vi "Periodic Tasks.vi"(8 "error in":errorcluster) -> ()   [LabVIEW 2017]
doc: "This VI runs in parallel to other tasks. It can contain as many user-defined periodic loops as you need. These can carry out PID or other sorts of timed response."
uses:
  <vilib>/Rock Robotics/WPI/Utilities/WPI_GetSetVariantRefNum.vi
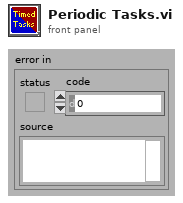
[diagram p1: front panel]
types:
  T1 = typedef "WPI_JoystickDevRef.ctl" = cluster{"Device":T2}
  T2 = typedef "WPI_JoystickDeviceEnum.ctl" = enum16{"USB 0", "USB 1", "USB 2", "USB 3", "USB 4", "USB 5"}
  T3 = typedef "WPI_MotorControlDeviceRef.ctl" = cluster{"DeviceStatus":errorcluster, "Type":T4, "PWM":cluster{"PWM Channel":T5, "DeadBand":T6}, "CAN":cluster{"Device Number":u8, "SetOutput VI Ref":variant, "GetOutput VI Ref":variant, "Enable VI Ref":variant, "Disable VI Ref":variant, "Data":variant}, "Invert":bool, "DIO PWM":cluster{"PWM \"Enable\" Channel":T5, "DIOChannel":T7, "PWM Rate":dbl}}
  T4 = typedef "WPI_MotorControlType.ctl" = enum16{"PWM", "CAN", "DIO PWM"}
  T5 = typedef "FPGA_DIOPWMChannel.ctl" = enum8{"PWM 0", "PWM 1", "PWM 2", "PWM 3", "PWM 4", "PWM 5", "PWM 6", "PWM 7", "PWM 8", "PWM 9", "PWM MXP 0", "PWM MXP 1", "PWM MXP 2", "PWM MXP 3", "PWM MXP 4", "PWM MXP 5", "PWM MXP 6", "PWM MXP 7", "PWM MXP 8", "PWM MXP 9", "Invalid"}
  T6 = typedef "WPI_PWMDeadband.ctl" = cluster{"Name":string, "maxPositivePwm":i32, "minPositivePwm":i32, "centerPwm":i32, "maxNegativePwm":i32, "minNegativePwm":i32, "angularRange":u16}
  T7 = typedef "FPGA_DIOChannel.ctl" = enum8{"DIO 0", "DIO 1", "DIO 2", "DIO 3", "DIO 4", "DIO 5", "DIO 6", "DIO 7", "DIO 8", "DIO 9", "DIO MXP 0", "DIO MXP 1", "DIO MXP 2", "DIO MXP 3", "DIO MXP 4", "DIO MXP 5", "DIO MXP 6", "DIO MXP 7", "DIO MXP 8", "DIO MXP 9", "DIO MXP 10", "DIO MXP 11", "DIO MXP 12", "DIO MXP 13", "DIO MXP 14", "DIO MXP 15", "SPI Port CS1", "SPI Port CS2", "SPI Port CS3", "SPI Port MISO", "SPI Port MOSI", "Invalid"}
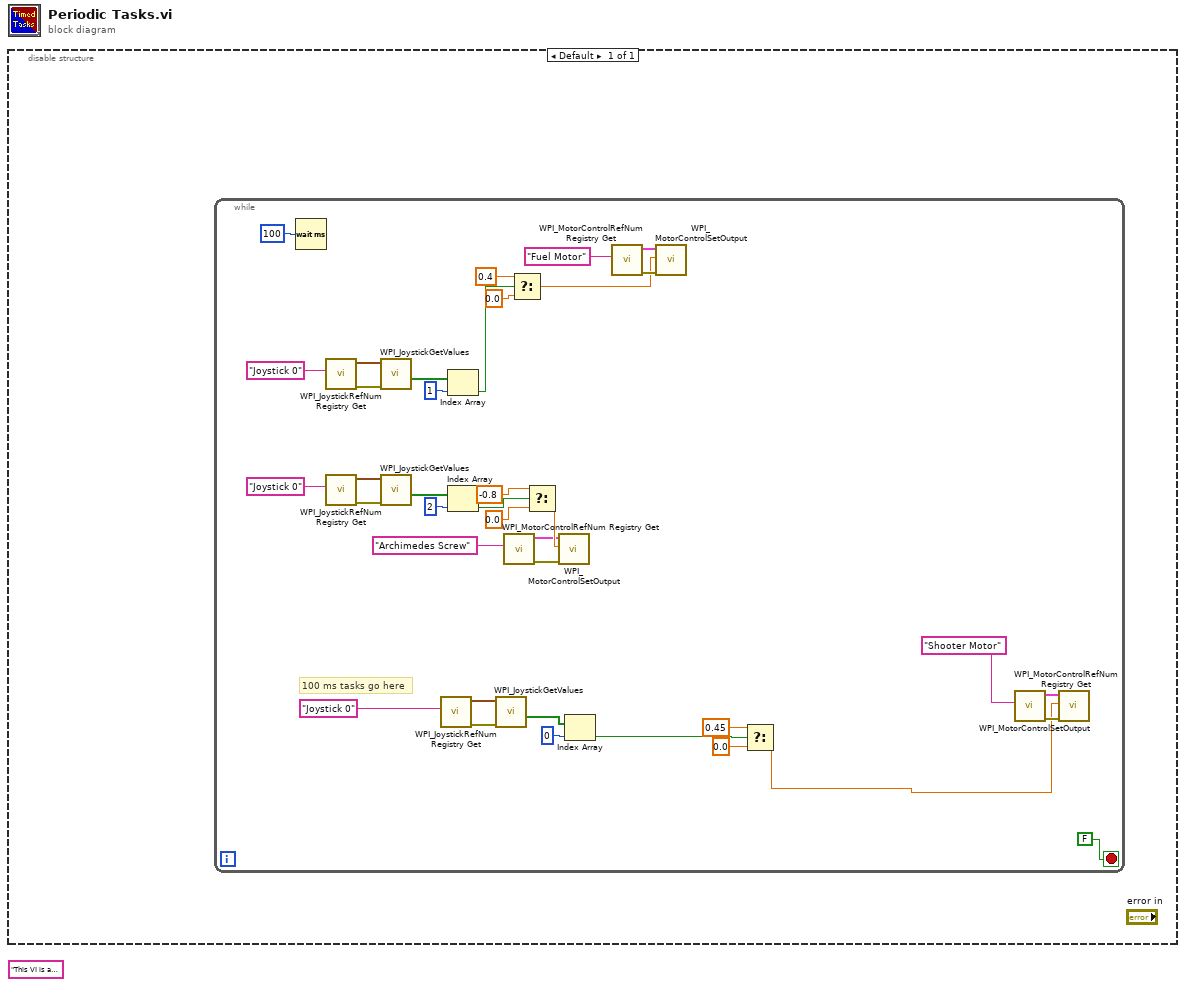
[diagram p0: block diagram]
diagram:
  (unwired) "This VI is a good place to take care of periodic tasks such as control loops.\n\nAdd code to the existing loops, or duplicate a loop to define a new rate. You can allocate I/O references here, or in Begin.vi.\n\nPeriodic loops will often operate with setpoints from other loops. Use a global variable such as Robot Global Data for sharing data between loops."
  n1 = disable-structure shown="Default" {
    frame Enabled {
      n2 = while {
        stop <- FALSE stop-if-true
        # "100 ms tasks go here"
        n3 = Wait (ms)(milliseconds to wait=u32 100) -> ()  [unwired: 1 out]
        n4 = call <vilib>:"WPI_JoystickRefNum Registry Get.vi"("refnum name"="Joystick 0") -> ("error out"=w25:errorcluster, "JoystickDevRef"=w24:T1)  [unwired: 9 in]
        n5 = call <vilib>:"WPI_JoystickRefNum Registry Get.vi"("refnum name"="Joystick 0") -> ("error out"=w26:errorcluster, "JoystickDevRef"=w27:T1)  [unwired: 9 in]
        n6 = call <vilib>:"WPI_JoystickGetValues.vi"("error in (no error)"=w25, "JoystickDevRef"=w24) -> ("Buttons"=w21:bool[])  [unwired: 5 in, 4 out]
        n7 = call <vilib>:"WPI_JoystickGetValues.vi"("error in (no error)"=w26, "JoystickDevRef"=w27) -> ("Buttons"=w30:bool[])  [unwired: 5 in, 4 out]
        n8 = call <vilib>:"WPI_JoystickRefNum Registry Get.vi"("refnum name"="Joystick 0") -> ("error out"=w10:errorcluster, "JoystickDevRef"=w11:T1)  [unwired: 9 in]
        n9 = Index Array(array=w21, index=1) -> (element=w18:bool)
        n10 = Index Array(array=w30, index=2) -> (element=w33:bool)
        n11 = call <vilib>:"WPI_JoystickGetValues.vi"("error in (no error)"=w10, "JoystickDevRef"=w11) -> ("Buttons"=w13:bool[])  [unwired: 5 in, 4 out]
        n12 = call <vilib>:"WPI_MotorControlRefNum Registry Get.vi"("refnum name"="Archimedes Screw") -> ("error out"=w28:errorcluster, "MotorControlDevRef"=w29:T3)  [unwired: 9 in]
        n13 = Select(t=0.4, s=w18, f=0.0) -> (s? t:f=w1:dbl)
        n14 = Select(t=-0.8, s=w33, f=0.0) -> (s? t:f=w35:dbl)
        n15 = call <vilib>:"WPI_MotorControlSetOutput.vi"("error in (no error)"=w28, "Output"=w35, "MotorControlDevRef"=w29) -> ()  [unwired: 6 in, 3 out]
        n16 = Index Array(array=w13, index=0) -> (element=w5:bool)
        n17 = call <vilib>:"WPI_MotorControlRefNum Registry Get.vi"("refnum name"="Fuel Motor") -> ("error out"=w23:errorcluster, "MotorControlDevRef"=w22:T3)  [unwired: 9 in]
        n18 = call <vilib>:"WPI_MotorControlSetOutput.vi"("error in (no error)"=w23, "Output"=w1, "MotorControlDevRef"=w22) -> ()  [unwired: 6 in, 3 out]
        n19 = Select(t=0.45, s=w5, f=0.0) -> (s? t:f=w6:dbl)
        n20 = call <vilib>:"WPI_MotorControlRefNum Registry Get.vi"("refnum name"="Shooter Motor") -> ("error out"=w8:errorcluster, "MotorControlDevRef"=w9:T3)  [unwired: 9 in]
        n21 = call <vilib>:"WPI_MotorControlSetOutput.vi"("error in (no error)"=w8, "Output"=w6, "MotorControlDevRef"=w9) -> ()  [unwired: 6 in, 3 out]
      }
    }
  }
